vi "No_fr_Alpha_Numeric_String.vi"(1 "Alpha Numeric String":string) -> (0 "Number":dbl format="%.2f")   [LabVIEW 2010]
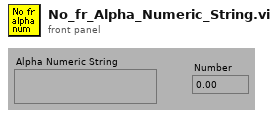
[diagram p1: front panel]
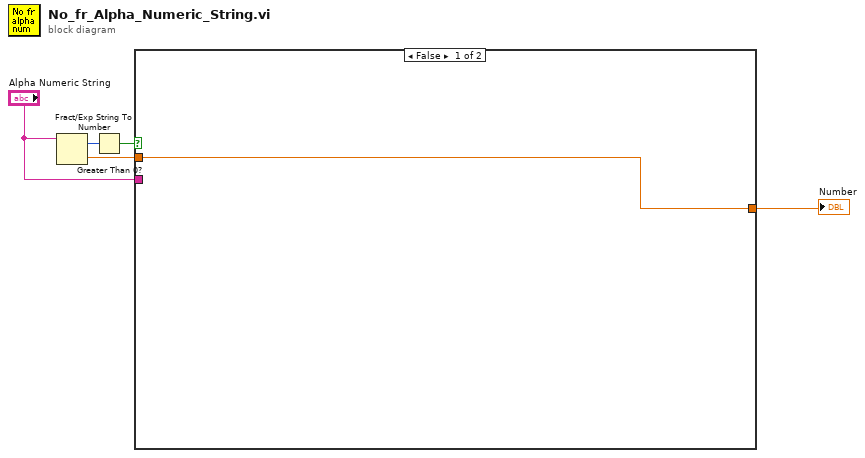
[diagram p0: block diagram]
diagram:
  n1 = Fract/Exp String To Number(string="Alpha Numeric String") -> (offset past number=w4:i32, number=w1:dbl)  [unwired: 3 in]
  n2 = Greater Than 0?(x=w4) -> (x > 0?=w3:bool)
  n3 = case shown="False" w3 {
    tunnel: "Alpha Numeric String" -> [_ _]
    tunnel: [w6 w7] -> w5
    tunnel: w1 -> [w6 w7]
    frame False {
    }
    frame True {
    }
  }
  "Number" <- w5
